vi "Cost.vi"(8 "error in (no error)":errorcluster, 11 "Abstract Beverage in":refnum<class "Abstract Beverage.lvclass">) -> (0 "error out":errorcluster, 2 "Cost":dbl, 3 "Abstract Beverage out":refnum<class "Abstract Beverage.lvclass">)   [LabVIEW 2013, in "Abstract Beverage.lvclass"]
uses:
  Abstract Beverage.lvclass
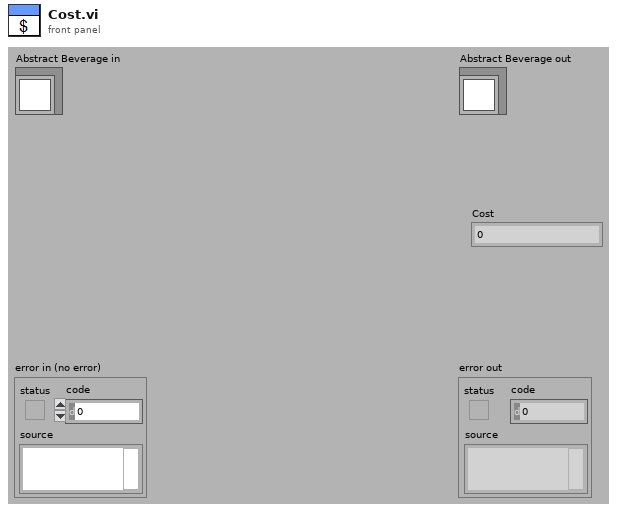
[diagram p1: front panel]
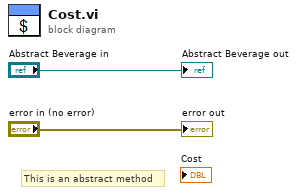
[diagram p0: block diagram]
diagram:
  # "This is an abstract method"
  "error out" <- "error in (no error)"
  "Abstract Beverage out" <- "Abstract Beverage in"
